vi "SaperaFrames2Vector.vi"() -> ()   [LabVIEW 2020]
uses:
  C:/Users/Opto/Downloads/GrabTestTDNI/GrabFrame4.dll
  Downloads/GrabTestTDNI/GrabFrame4.dll
  C:/Users/Opto/Desktop/Equipamentos/SaperaFrames2Vector/DALSA.SaperaLT.SapClassBasic.dll
  DALSA.SaperaLT.SapClassBasic.dll
panel:
  out "Snap Create:":bool
  out "Buffer Create:":bool
  out "Xfer Create:":bool
  out "Elapsed Time (seconds):":dbl caption="Elapsed Time (s)"
  in  "Number of frames:":i32=3
  out "error SaveFrame":errorcluster
  out "error final":errorcluster
  out "error sapTransfer Dispose":errorcluster
  out "countFrame":i32
  out "Wait Transfer:":bool
  out "Destroy Objects:":bool
  out "Frames Array:":i16[][](array[numeric])
  out "File Opened:":bool
  out "File path:":string="C:\\temp\\IC-47_TDI.ccf"
  # "Camera's File Configuration (.ccf):"
  # "Indicators flags of control:"
  # "Results:"
  # "Debug info:"
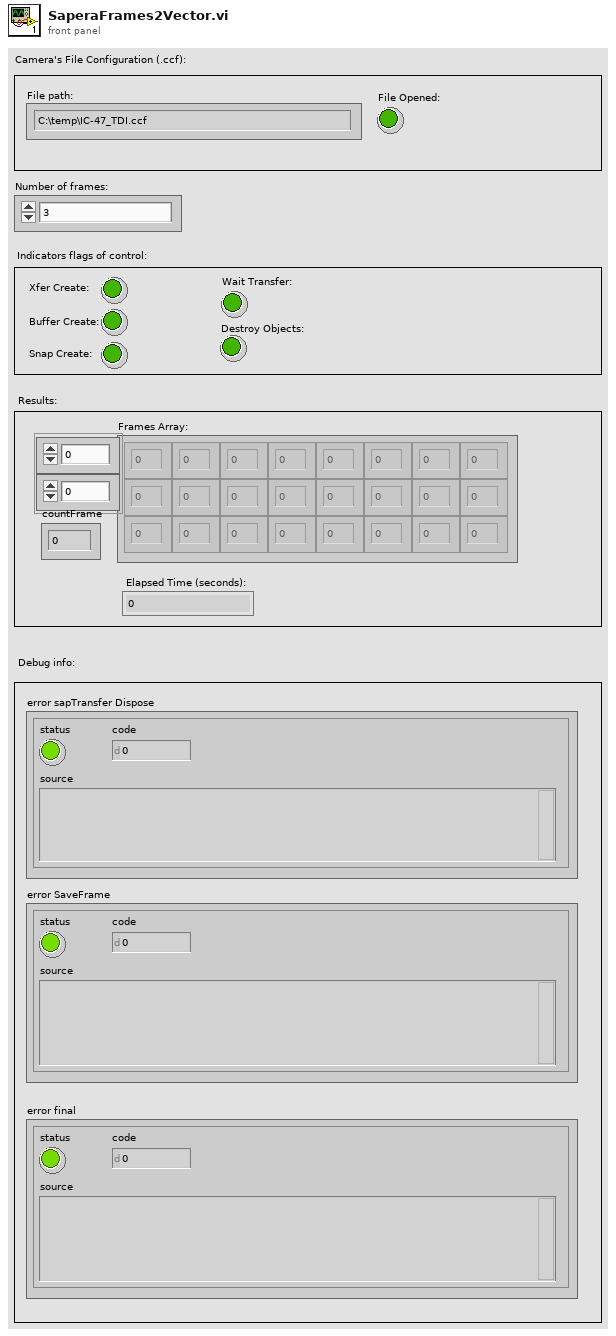
[diagram p1: front panel]
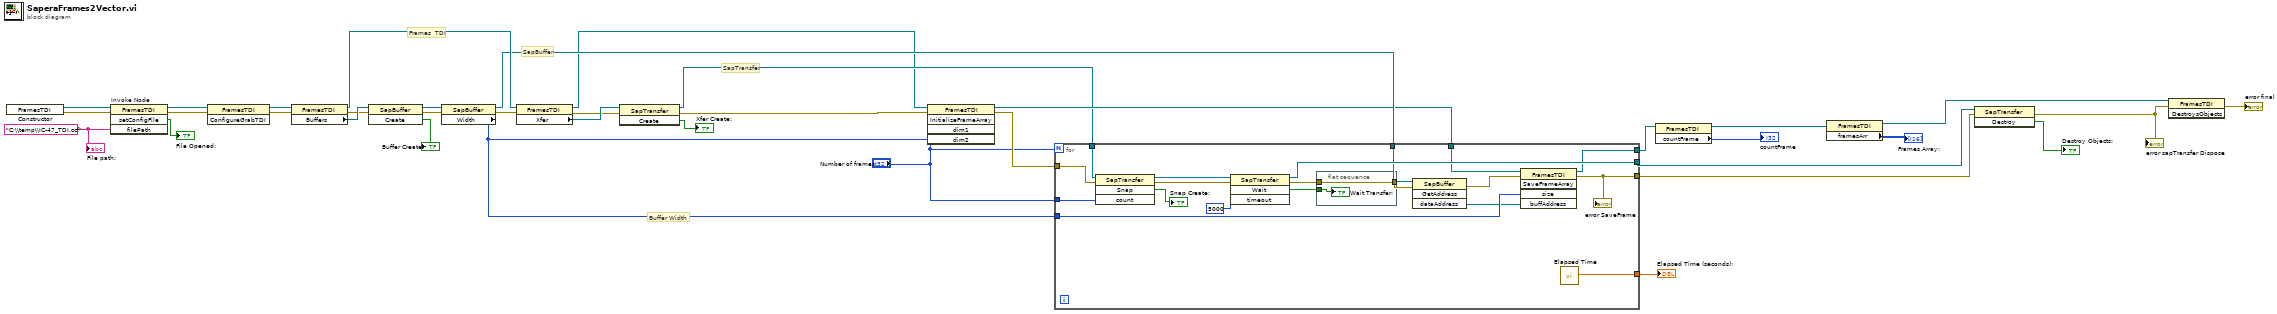
[diagram p0: block diagram]
diagram:
  w33 = "C:\\temp\\IC-47_TDI.ccf" ("filePath")
  # "Buffer Width"
  # "SapTransfer"
  # "SapBuffer"
  # "Frames  TDI"
  n1 = constructor class="FramesTDI"() -> (reference out=w36:refnum<k24>, error out=w37:errorcluster)  [unwired: 3 in, 1 out]
  n2 = invoke on="Invoke Node" class="FramesTDI" method="setConfigFile"(reference=w36, error in=w37, "filePath"=w33) -> (reference out=w35:refnum<k24>, error out=w34:errorcluster, "setConfigFile"=→"File Opened:":bool)  [unwired: 1 in, 1 out]
  n3 = invoke class="FramesTDI" method="ConfigureGrabTDI"(reference=w35, error in=w34) -> (reference out=w31:refnum<k24>, error out=w27:errorcluster)  [unwired: 1 in, 1 out]
  n4 = property class="FramesTDI"(reference=w31, error in=w27) -> (reference out=w22:refnum<k24>, error out=w26:errorcluster, "Buffers"=w30:refnum<k24>)
  n5 = invoke class="SapBuffer" method="Create"(reference=w30, error in=w26) -> (reference out=w28:refnum<k24>, error out=w25:errorcluster, "Create"=→"Buffer Create:":bool)  [unwired: 1 in]
  n6 = property class="SapBuffer"(reference=w28, error in=w25) -> (reference out=w17:refnum<k24>, error out=w24:errorcluster, "Width"=w15:i32)
  n7 = property class="FramesTDI"(reference=w22, error in=w24) -> (reference out=w5:refnum<k24>, error out=w23:errorcluster, "Xfer"=w29:refnum<k24>)
  n8 = invoke class="SapTransfer" method="Create"(reference=w29, error in=w23) -> (reference out=w10:refnum<k24>, error out=w4:errorcluster, "Create"=→"Xfer Create:":bool)  [unwired: 1 in]
  n9 = invoke class="FramesTDI" method="InitializeFrameArray"(reference=w5, error in=w4, "dim1"="Number of frames:", "dim2"=w15) -> (reference out=w16:refnum<k24>, error out=w19:errorcluster)  [unwired: 1 in, 3 out]
  n10 = for {
    N: "Number of frames:" -> [_]
    tunnel: w10 -> [w56]
    tunnel: w19 -> [w55]
    tunnel: "Number of frames:" -> [w54]
    tunnel: [w51] -> w18
    tunnel: w17 -> [w47]
    tunnel: w16 -> [w45]
    tunnel: w15 -> [w43]
    tunnel: [w41] -> w12
    tunnel: [w40] -> w14
    tunnel: [w39] -> w3
    n11 = invoke class="SapTransfer" method="Snap"(reference=w56, error in=w55, "count"=w54) -> (reference out=w53:refnum<k24>, error out=w52:errorcluster, "Snap"=→"Snap Create:":bool)  [unwired: 1 in, 1 out]
    n12 = invoke class="SapTransfer" method="Wait"(reference=w53, error in=w52, "timeout"=5000) -> (reference out=w51:refnum<k24>, error out=w48:errorcluster, "Wait"=w49:bool)  [unwired: 1 in, 1 out]
    n13 = flat-sequence {
      tunnel: w49 -> [w58]
      tunnel: w48 -> [w57]
      tunnel: [w57] -> w46
      frame #0 {
        "Wait Transfer:" <- w58
      }
    }
    n14 = invoke class="SapBuffer" method="GetAddress"(reference=w47, error in=w46) -> (error out=w44:errorcluster, "dataAddress"=w42:refnum<k24>)  [unwired: 2 in, 2 out]
    n15 = invoke class="FramesTDI" method="SaveFrameArray"(reference=w45, error in=w44, "size"=w43, "buffAddress"=w42) -> (reference out=w41:refnum<k24>, error out=w40:errorcluster)  [unwired: 1 in, 3 out]
    "error SaveFrame" <- w40
    n16 = call "Elapsed Time"() -> ("Elapsed Time (s)"=w39:dbl)  [unwired: 12 in, 7 out]
  }
  "Elapsed Time (seconds):" <- w3
  n17 = property class="FramesTDI"(reference=w12) -> (reference out=w13:refnum<k24>, "countFrame"=→"countFrame":i32)  [unwired: 1 in, 1 out]
  n18 = property class="FramesTDI"(reference=w13) -> (reference out=w9:refnum<k24>, "framesArr"=→"Frames Array:":i16[][])  [unwired: 1 in, 1 out]
  n19 = invoke class="SapTransfer" method="Destroy"(reference=w18, error in=w14) -> (error out=w7:errorcluster, "Destroy"=→"Destroy Objects:":bool)  [unwired: 1 in, 1 out]
  "error sapTransfer Dispose" <- w7
  n20 = invoke class="FramesTDI" method="DestroysObjects"(reference=w9, error in=w7) -> (error out=→"error final":errorcluster)  [unwired: 1 in, 2 out]
  "File path:" <- w33
